vi "Main.vi"() -> ()   [LabVIEW 2015, in "Device Under Test_Cloneable_DQMH.lvlib"]
doc: "This application is based on the Delacor QMH project template. Run this VI directly to test the module in stand alone mode. Run the module tester VI to test the module in external launch mode.\n\nThis example implements a Device Under Test with a cloneable Delacor QMH module.\n_____\nBased on Delacor QMH Project Template 2.0.0.62.\nReviewed and updated to match QMH Project Template 4.0.\n<b>Note:</b> This VI was modified by the <b>Validate DQMH Module</b> tool to upgrade it to the DQMH 3.0 implementation of the 'Show Diagram' message, which checks the password-protected status of the Main VI before showing the diagram.\n____\nDelacor QMH Thermal Chamber Examples 4.0.0.21\nCopyright (c) 2018, Delacor"
uses:
  Device Under Test_Cloneable_DQMH.lvlib
  <vilib>/Delacor/Delacor QMH/Libraries/Cloneable Module Admin_class/Delacor_lib_QMH_Cloneable Module Admin.lvclass
  Module Data--cluster.ctl
  GUI Control References--cluster.ctl
  Set Power State Argument--cluster.ctl
  <vilib>/Delacor/Delacor QMH/Libraries/Cloneable Module Admin_class/Delacor_lib_QMH_Cloneable Module Admin.lvclass/Delacor_lib_QMH_Cloneable Module Admin.ctl
  Perform Self Test Argument--cluster.ctl
  Perform Self Test (Reply Payload)--cluster.ctl
  Update DUT Status Argument--cluster.ctl
  Stop Argument--cluster.ctl
  <vilib>/Delacor/Delacor QMH/Libraries/Module Admin_class/Delacor_lib_QMH_Module Admin.lvclass/Delacor_lib_QMH_Module Admin.ctl
  <vilib>/Delacor/Delacor QMH/Libraries/Cloneable Module Admin_class/Delacor_lib_QMH_Get Module ID.vi
  <vilib>/Delacor/Delacor QMH/Libraries/Module Admin_class/Delacor_lib_QMH_Get External Launch.vi
  <vilib>/Delacor/Delacor QMH/Libraries/Message Queue_class/Delacor_lib_QMH_Enqueue Message (Single).vi
  <vilib>/Utility/error.llb/Error Cluster From Error Code.vi
  <vilib>/ErrorRing/Error Ring.xnode
  <vilib>/Delacor/Delacor QMH/Libraries/Message Queue_class/Delacor_lib_QMH_Message Queue.lvclass
  Clone Registration/Clone Registration.lvlib
panel:
  in  "Self Test":bool
  in  "Power Off":bool
  in  "Power On":bool
  out "Self Test Result":bool
  out "Power  State":bool
  out "error out":errorcluster
  in  "Module Admin":refnum<class "Delacor_lib_QMH_Cloneable Module Admin.lvclass">
  out "Status":string
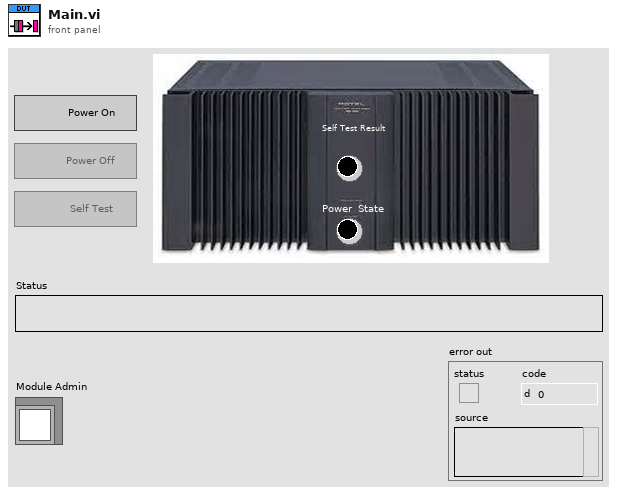
[diagram p1: front panel]
types:
  T1 = typedef "Device Under Test_Cloneable_DQMH.lvlib/Request Events--cluster.ctl" = cluster{"Stop Module":refnum<user-event>, "Show Panel":refnum<user-event>, "Hide Panel":refnum<user-event>, "Show Diagram":refnum<user-event>, "Set Power State":refnum<user-event>, "Perform Self Test":refnum<user-event>, "Update DUT Status":refnum<user-event>, "Get Module Execution Status":refnum<user-event>}
  T2 = typedef "Device Under Test_Cloneable_DQMH.lvlib/Module Data--cluster.ctl" = cluster{"Status":string, "Power State":bool, "Self Test Result":bool, "References":T3}
  T3 = typedef "Device Under Test_Cloneable_DQMH.lvlib/GUI Control References--cluster.ctl" = cluster{"Power On Button":refnum<vi>, "Power Off Button":refnum<vi>, "Self Test Button":refnum<vi>, "Power State LED":refnum<vi>, "Self Test Result LED":refnum<vi>}
  T4 = typedef "Device Under Test_Cloneable_DQMH.lvlib/Set Power State Argument--cluster.ctl" = cluster{"Module ID":i32, "Power State":bool}
  T5 = typedef "Device Under Test_Cloneable_DQMH.lvlib/Perform Self Test Argument--cluster.ctl" = cluster{"Module ID":i32, "Wait Notifier":refnum<notifier>}
  T6 = typedef "Device Under Test_Cloneable_DQMH.lvlib/Update DUT Status Argument--cluster.ctl" = cluster{"Module ID":i32, "Self Test Result":bool, "Power State":bool}
  T7 = enum32{"invalid lock state", "Not Locked", "Locked (No Password)", "Password-protected"}
  T8 = typedef "Device Under Test_Cloneable_DQMH.lvlib/Stop Argument--cluster.ctl" = cluster{"Origin":string, "Module ID":i32, "Exit via Stop Module Req?":bool, "Wait for Module to stop?":bool}
  T9 = enum32{"Invalid", "Standard", "Closed", "Hidden", "Minimized", "Maximized"}
  T10 = typedef "Device Under Test_Cloneable_DQMH.lvlib/Perform Self Test (Reply Payload)--cluster.ctl" = cluster{"Result":bool, "error":errorcluster}
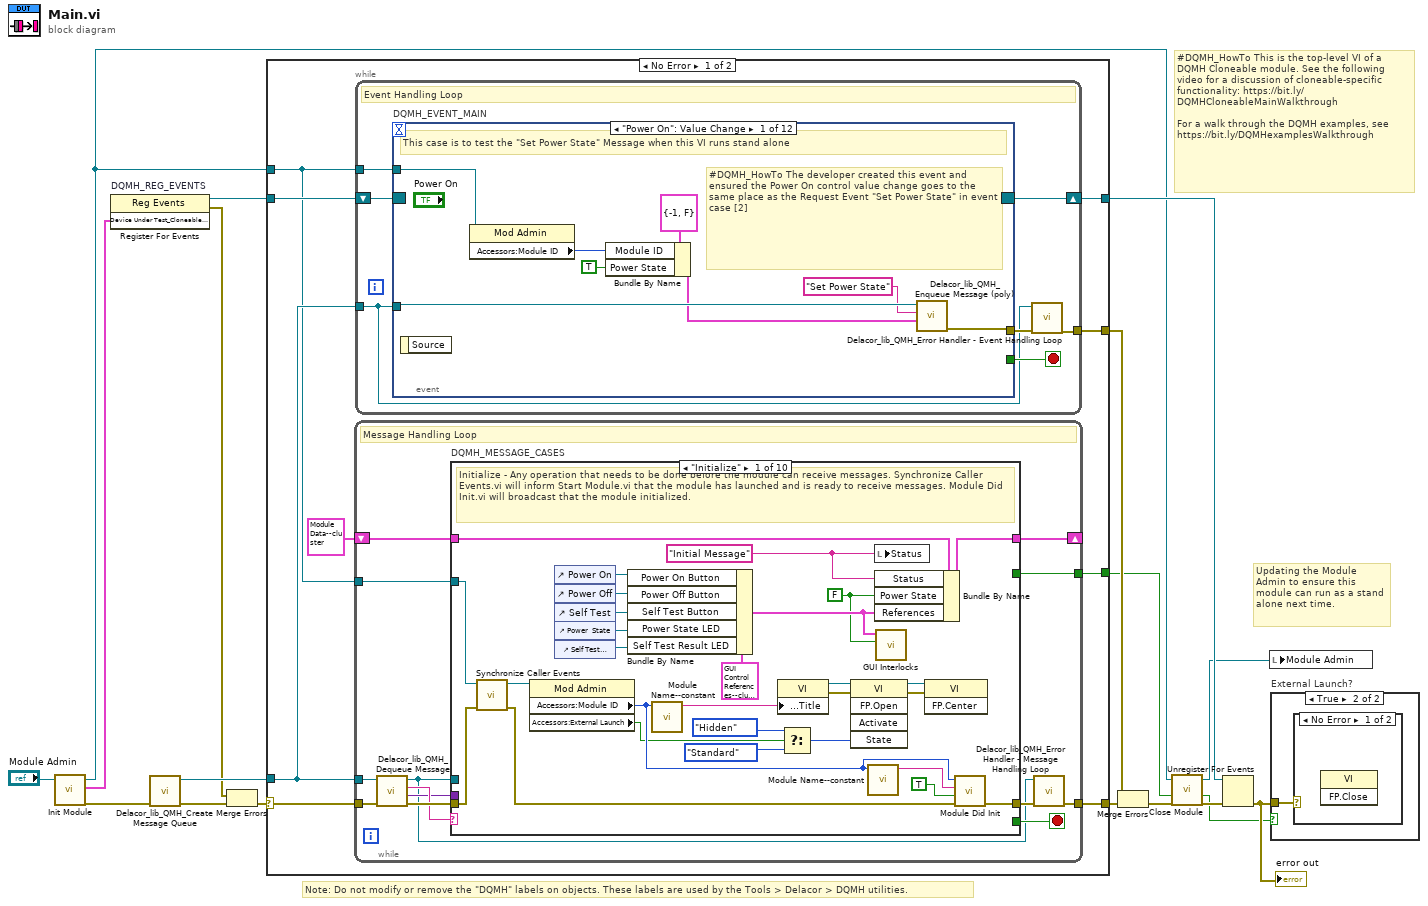
[diagram p0: block diagram]
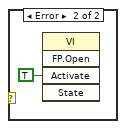
[diagram p3: hidden frame]
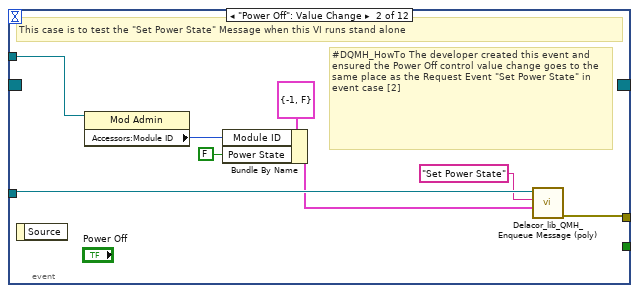
[diagram p4: hidden frame]
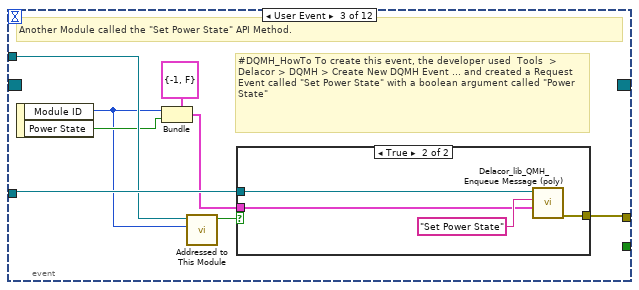
[diagram p5: hidden frame]
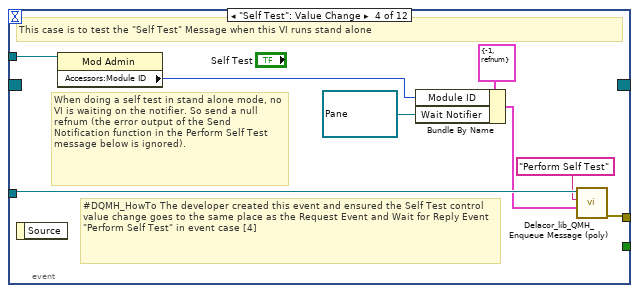
[diagram p7: hidden frame]
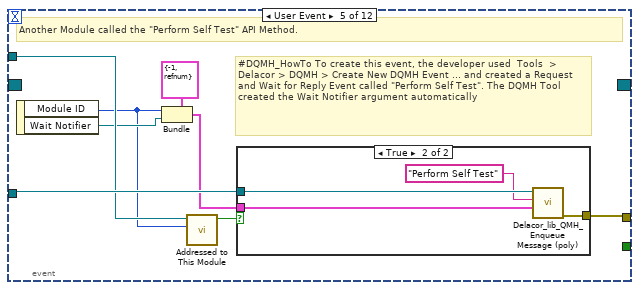
[diagram p8: hidden frame]
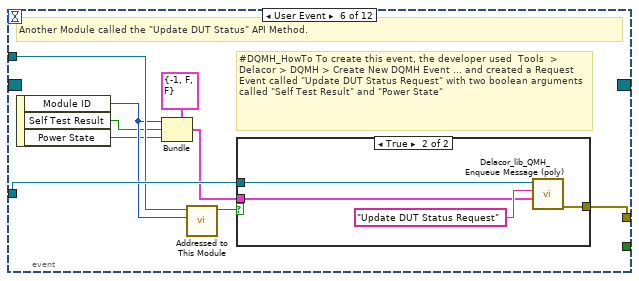
[diagram p10: hidden frame]
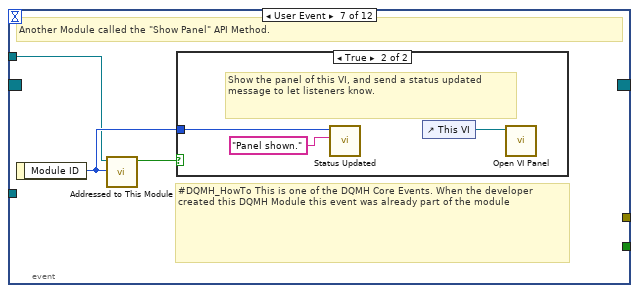
[diagram p12: hidden frame]
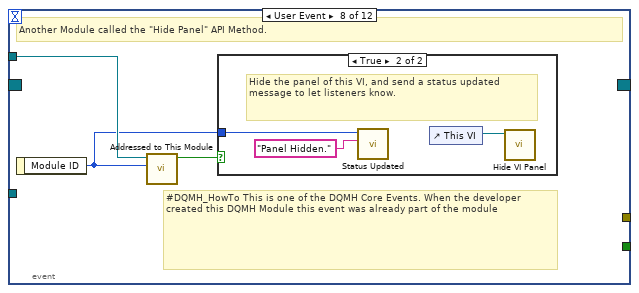
[diagram p14: hidden frame]
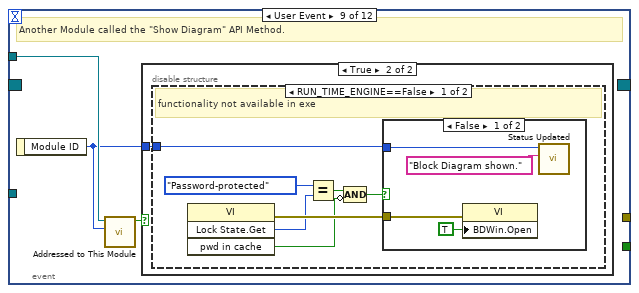
[diagram p16: hidden frame]
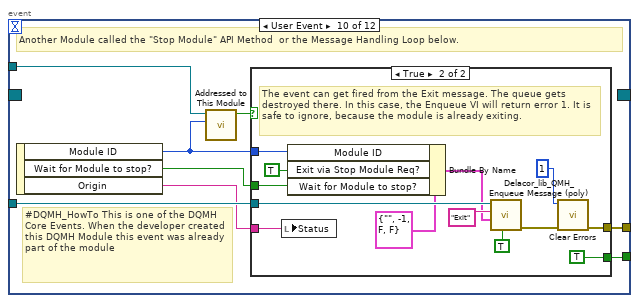
[diagram p20: hidden frame]
diagram:
  # "#DQMH_HowTo This is the top-level VI of a DQMH Cloneable module. See the following video for a discussion of cloneable-specific functionality: https://bit.ly/DQMHCloneableMainWalkthrough\n\nFor a walk through the DQMH examples, see https://bit.ly/DQMHexamplesWalkthrough"
  # "Note: Do not modify or remove the \"DQMH\" labels on objects. These labels are used by the Tools > Delacor > DQMH utilities."
  # "Updating the Module Admin to ensure this module can run as a stand alone next time."
  n1 = call "Init Module.vi"("Cloneable Module Admin in"="Module Admin") -> ("error out"=w15:errorcluster, "Device Under Test_Cloneable_DQMH Request Events"=w12:T1, "Cloneable Module Admin out"=w8:refnum<class "Delacor_lib_QMH_Cloneable Module Admin.lvclass">)  [unwired: 8 in]
  n2 = register-events "DQMH_REG_EVENTS"(w12) -> (reference out=w13:refnum<event-registration>, error out=w1:errorcluster)  [unwired: 2 in]
  n3 = call <vilib>:"Delacor_lib_QMH_Create Message Queue.vi"("error in (no error)"=w15) -> ("error out"=w3:errorcluster, "Message Queue out"=w11:refnum<class "Delacor_lib_QMH_Message Queue.lvclass">)  [unwired: 9 in]
  n4 = Merge Errors(w1, w3) -> (w2:errorcluster)
  n5 = case shown="No Error" w2 {
    selector: w2 -> [w21 w320]
    tunnel: [w27 w320] -> w16
    tunnel: [w26 w321] -> w14
    tunnel: w13 -> [w24 w321]
    tunnel: w11 -> [w23 _]
    tunnel: [w22 _] -> w17
    tunnel: w8 -> [w20 w316]
    tunnel: [w19 _] -> w6
    frame No Error {
      n6 = while {
        tunnel: w23 -> [w165]
        shift-right: [w171] -> _
        shift-left: T2 {"Status"="", "Power State"=FALSE, "Self Test Result"=FALSE, "References"={"Power On Button"=refnum, "Power Off Button"=refnum, "Self Test Button"=refnum, "Power State LED"=refnum, "Self Test Result LED"=refnum}} ("Data Cluster") -> [w172]
        tunnel: w21 -> [w169]
        tunnel: [w163] -> w27
        tunnel: w20 -> [w162]
        tunnel: [w161] -> w19
        stop <- w170 stop-if-true
        # "Message Handling Loop"
        n7 = call-dynamic "Delacor_lib_QMH_Dequeue Message.vi"("error in (no error)"=w169, "Message Queue in"=w165) -> ("error out"=w168:errorcluster, "Message Data"=w166:variant, "Message"=w167:string, "Message Queue out"=w164:refnum<class "Delacor_lib_QMH_Message Queue.lvclass">)  [unwired: 6 in]
        n8 = case "DQMH_MESSAGE_CASES" shown="\"Initialize\"" w167 {
          selector: w167 -> [_ _ _ _ _ _ _ _ _ w303]
          tunnel: w164 -> [_ _ _ w228 w239 w251 _ w267 w297 _]
          tunnel: w168 -> [w193 w214 w216 w230 w246 w264 w266 w277 w299 _]
          tunnel: [w186 w206 w216 w220 w231 w252 w266 w272 w293 w304] -> w173
          tunnel: w172 -> [w192 w205 w215 w227 w235 w263 w265 w276 w296 w305]
          tunnel: [w191 w205 w215 w224 w242 w263 w265 w276 w296 w305] -> w171
          tunnel: [_ _ _ _ _ _ _ _ w295 _] -> w170
          tunnel: w166 -> [_ w213 _ w217 w238 w262 _ w275 w289 _]
          tunnel: w162 -> [w183 w209 _ _ _ _ _ w271 w285 w301]
          tunnel: [_ _ _ _ _ _ _ _ w287 _] -> w161
          frame "Initialize" {
            w174 = FALSE ("Power State")
            w190 = "Initial Message" ("Initial Message")
            # "Initialize - Any operation that needs to be done before the module can receive messages. Synchronize Caller Events.vi will inform Start Module.vi that the module has launched and is ready to receive messages. Module Did Init.vi will broadcast that the module initialized."
            n9 = call "Synchronize Caller Events.vi"("error in (no error)"=w193, "Module Admin"=w183) -> ("error out"=w187:errorcluster, "Module Admin out"=w182:refnum<class "Delacor_lib_QMH_Cloneable Module Admin.lvclass">)  [unwired: 8 in]
            n10 = property class="Mod Admin"(reference=w182) -> ("Accessors:Module ID"=w185:i32, "Accessors:External Launch"=w184:bool)  [unwired: 1 in, 2 out]
            n11 = control-ref of="Power On"() -> (w180:refnum<vi>)
            n12 = control-ref of="Power Off"() -> (w179:refnum<vi>)
            n13 = control-ref of="Self Test"() -> (w178:refnum<vi>)
            n14 = control-ref of="Power  State"() -> (w177:refnum<vi>)
            n15 = control-ref of="Self Test Result"() -> (w176:refnum<vi>)
            n16 = Bundle By Name(cluster=T3 {"Power On Button"=refnum, "Power Off Button"=refnum, "Self Test Button"=refnum, "Power State LED"=refnum, "Self Test Result LED"=refnum} ("References"), "Power On Button"=w180, "Power Off Button"=w179, "Self Test Button"=w178, "Power State LED"=w177, "Self Test Result LED"=w176) -> (w175:T3)
            n17 = call "Module Name--constant.vi"("Module ID"=w185) -> ("Module Name"=w197:string)  [unwired: 10 in]
            n18 = property class="VI"("Front Panel.Title"=w197) -> (reference out=w200:refnum<vi>, error out=w201:errorcluster)  [unwired: 2 in]
            n19 = Select(t=T9."Hidden" ("State"), s=w184, f=T9."Standard" ("State")) -> (s? t:f=w194:T9)
            n20 = invoke class="VI" method="FP.Open"(reference=w200, error in=w201, "State"=w194) -> (reference out=w199:refnum<vi>, error out=w198:errorcluster)  [unwired: 2 in, 3 out]
            n21 = call "Module Name--constant.vi"("Module ID"=w185) -> ("Module Name"=w188:string)  [unwired: 10 in]
            n22 = local write "Status"(w190) -> ()
            n23 = Bundle By Name(cluster=w192, "Status"=w190, "Power State"=w174, "References"=w175) -> (w191:T2)
            n24 = call "GUI Interlocks.vi"("Power State"=w174, "References"=w175) -> ()  [unwired: 10 in]
            n25 = invoke class="VI" method="FP.Center"(reference=w199, error in=w198) -> ()  [unwired: 1 in, 3 out]
            n26 = call "Module Did Init.vi"("error in (no error)"=w187, "Initialized?"=TRUE, "Origin"=w188, "Module ID"=w185) -> ("error out"=w186:errorcluster)  [unwired: 7 in]
          }
          frame "Update Display" {
            # "Update Display - Update user interface here."
            n27 = property class="Mod Admin"(reference=w209) -> ("Accessors:Module ID"=w208:i32)  [unwired: 1 in, 2 out]
            n28 = Variant To Data(error in=w214, type="", Variant=w213) -> (data=w211:string, error out=w210:errorcluster)
            "Status" <- w211
            n29 = Unbundle By Name(w205) -> ("References"=w204:T3, "Power State"=w203:bool, "Self Test Result"=w202:bool)
            "Power  State" <- w203
            "Self Test Result" <- w202
            n30 = call "Status Updated.vi"("error in (no error)"=w210, "Status"=w211, "Module ID"=w208) -> ("error out"=w207:errorcluster)  [unwired: 8 in]
            n31 = call "GUI Interlocks.vi"("Power State"=w203, "References"=w204) -> ()  [unwired: 10 in]
            n32 = call "DUT Status Updated.vi"("error in (no error)"=w207, "Self Test Result"=w202, "Power State"=w203, "Module ID"=w208) -> ("error out"=w206:errorcluster)  [unwired: 7 in]
          }
          frame "---DUT---" {
            # "Separator - The following cases handle DUT specific messages."
          }
          frame "Set Power State" {
            # "#DQMH_HowTo To create this case, the developer used  Tools  > Delacor > DQMH > Create New DQMH Event ... and created a Request Event called \"Set Power State\" with a boolean argument called \"Power State\""
            # "Update the power state of the DUT. Broadcast a message that the power state was updated."
            n33 = Variant To Data(error in=w230, type=T4 {"Module ID"=-1, "Power State"=FALSE} ("Set Power State Argument"), Variant=w217) -> (data=w225:T4, error out=w229:errorcluster)
            n34 = Unbundle By Name(w225) -> ("Power State"=w219:bool)
            n35 = Format Into String(format string="DUT Power State Set to %s", w219) -> (resulting string=w221:string)  [unwired: 2 in, 1 out]
            n36 = Bundle By Name(cluster=w227, "Power State"=w219, "Self Test Result"=FALSE) -> (w224:T2)
            n37 = call-poly <vilib>:"Delacor_lib_QMH_Enqueue Message (poly).vi"("error in (no error)"=w229, "Message Data"=w221, "Message"="Update Display", "Message Queue in"=w228) -> ("error out"=w220:errorcluster)  [unwired: 6 in, 1 out]
          }
          frame "Perform Self Test" {
            # "#DQMH_HowTo To create this case, the developer used  Tools  > Delacor > DQMH > Create New DQMH Event ... and created a Request Event and Wait for Reply called \"Perform Self Test\" without arguments"
            # "Perform a self test of the DUT. Update the display with the result, and broadcast a message indicating the result of the self test."
            n38 = Unbundle By Name(w235) -> ("Power State"=w234:bool)
            n39 = Variant To Data(error in=w246, type=T5 {"Module ID"=-1, "Wait Notifier"=refnum} ("Perform Self Test Argument"), Variant=w238) -> (data=w244:T5, error out=w232:errorcluster)
            n40 = Unbundle By Name(w244) -> ("Wait Notifier"=w243:refnum<notifier>)
            n41 = case shown="True" w234 {
              tunnel: [_ w249] -> w236
              tunnel: ["DUT is powered off, cannot perform self test." ("format string") w248] -> w233
              frame False {
              }
              frame True {
                n42 = call "Simulate Self Test.vi"() -> ("Result"=w249:bool)  [unwired: 11 in]
                n43 = Format Into String(format string="DUT Self Test Result: %s", w249) -> (resulting string=w248:string)  [unwired: 2 in, 1 out]
              }
            }
            n44 = Bundle By Name(cluster=T10 {"Result"=FALSE, "error"={"status"=FALSE, "code"=0, "source"=""}} ("notification"), "Result"=w236, "error"=w232) -> (w240:T10)
            n45 = Bundle By Name(cluster=w235, "Self Test Result"=w236) -> (w242:T2)
            n46 = Send Notification(notification=w240, notifier=w243) -> ()  [unwired: 1 in, 2 out]
            n47 = call-poly <vilib>:"Delacor_lib_QMH_Enqueue Message (poly).vi"("error in (no error)"=w232, "Message Data"=w233, "Message"="Update Display", "Message Queue in"=w239) -> ("error out"=w231:errorcluster)  [unwired: 6 in, 1 out]
          }
          frame "Update DUT Status Request" {
            # "#DQMH_HowTo To create this case, the developer used  Tools  > Delacor > DQMH > Create New DQMH Event ... and created a Request Event called \"Update DUT Status Request\" with two boolean arguments called \"Self Test Result\" and \"Power State\""
            # "Read the state of the DUT and broadcast it."
            n48 = Variant To Data(error in=w264, type=T6 {"Module ID"=-1, "Self Test Result"=FALSE, "Power State"=FALSE} ("Update DUT Status Request Argument"), Variant=w262) -> (data=w260:T6, error out=w256:errorcluster)
            n49 = Unbundle By Name(w260) -> ("Module ID"=w259:i32, "Self Test Result"=w258:bool, "Power State"=w257:bool)
            n50 = call "DUT Status Updated.vi"("error in (no error)"=w256, "Self Test Result"=w257, "Power State"=w258, "Module ID"=w259) -> ("error out"=w253:errorcluster)  [unwired: 7 in]
            n51 = call-poly <vilib>:"Delacor_lib_QMH_Enqueue Message (poly).vi"("error in (no error)"=w253, "Message Data"="DUT Status Updated" ("format string"), "Message"="Update Display", "Message Queue in"=w251) -> ("error out"=w252:errorcluster)  [unwired: 6 in, 1 out]
          }
          frame "---Exit and Error Handling---" {
            # "Separator - The following cases handle error and exit messages."
          }
          frame "Error" {
            # "#DQMH_HowTo When the developer created this DQMH Module this case was already part of the module"
            # "Error - Check the error message data and respond accordingly. This message is sent by the \"Error Handler\" VIs at the end of each loop in this application."
            n52 = property class="Mod Admin"(reference=w271) -> ("Accessors:External Launch"=w268:bool, "Accessors:Module ID"=w270:i32)  [unwired: 1 in, 2 out]
            n53 = Variant To Data(error in=w277, type=errorcluster {"status"=FALSE, "code"=0, "source"=""} ("error constant"), Variant=w275) -> (data=w278:errorcluster, error out=w273:errorcluster)
            n54 = call "Error Reported.vi"("Error"=w278, "Module ID"=w270) -> ()  [unwired: 9 in, 1 out]
            n55 = case shown="False" w268 {
              tunnel: [w283 _] -> w269
              tunnel: w267 -> [w282 _]
              tunnel: w278 -> [w279 _]
              frame False {
                # "If the module is running standalone, then pop up an error dialog and call the \"Exit\" message."
                n56 = call <vilib>:"Simple Error Handler.vi"("error in (no error)"=w279) -> ()  [unwired: 4 in, 5 out]
                n57 = call-poly <vilib>:"Delacor_lib_QMH_Enqueue Message (poly).vi"("Priority Message? (F)"=TRUE, "Message"="Exit", "Message Queue in"=w282) -> ("error out"=w283:errorcluster)  [unwired: 7 in, 1 out]
              }
              frame True {
                # "If the module was launched externally, calling the Error Reported broadcast VI is the only action performed by the \"Error\" message. The module's caller can then process the error appropriately."
              }
            }
            n58 = Merge Errors(w273, w269) -> (w272:errorcluster)
          }
          frame "Exit" {
            w291 = 91  # 91: not all Exit messages will have an argument
            w295 = TRUE  # Stop the VI
            # "#DQMH_HowTo When the developer created this DQMH Module this case was already part of the module"
            # "Release the message queue reference"
            # "Exit - Exit the application."
            n59 = Variant To Data(error in=w299, type=T8 {"Origin"="", "Module ID"=-1, "Exit via Stop Module Req?"=FALSE, "Wait for Module to stop?"=FALSE} ("Stop Argument"), Variant=w289) -> (data=w286:T8, error out=w290:errorcluster)
            n60 = call <vilib>:"Clear Errors.vi"("error in (no error)"=w290, "specific error code to clear (0: all)"=w291) -> ("error out"=w298:errorcluster)  [unwired: 4 in, 1 out]
            n61 = control-ref of="This VI"() -> (w284:refnum<vi>)
            n62 = call-dynamic "Delacor_lib_QMH_Release Message Queue.vi"("error in (no error)"=w298, "Message Queue"=w297) -> ("error out"=w294:errorcluster)  [unwired: 9 in]
            n63 = call "Handle Exit.vi"("Stop Argument"=w286, "Module Admin in"=w285, "VI reference"=w284) -> ("error out"=w292:errorcluster, "Wait for Stop?"=w287:bool)  [unwired: 7 in]
            n64 = Merge Errors(w292, w294) -> (w293:errorcluster)
          }
          frame Default {
            # "#DQMH_HowTo When the developer created this DQMH Module this case was already part of the module"
            # "'Default' case only runs if there is a message that isn't defined in any of the other cases.  Output a programming error."
            n65 = property class="Mod Admin"(reference=w301) -> ("Accessors:Module ID"=w300:i32)  [unwired: 1 in, 2 out]
            n66 = call "Module Name--constant.vi"("Module ID"=w300) -> ("Module Name"=w302:string)  [unwired: 10 in]
            n67 = xnode "Error Ring"("parameter 0"=w303, "parameter 1"=w302) -> ("error out"=w304:errorcluster)
          }
        }
        n68 = call-dynamic "Delacor_lib_QMH_Error Handler - Message Handling Loop.vi"("error in (no error)"=w173, "Message Queue in"=w164) -> ("dup error in"=w163:errorcluster)  [unwired: 8 in, 1 out]
      }
      n69 = while {
        tunnel: w23 -> [w28]
        shift-right: [w33] -> w26
        shift-left: w24 -> [w34]
        tunnel: [w30] -> w22
        tunnel: w20 -> [w29]
        stop <- w31 stop-if-true
        # "Event Handling Loop"
        n70 = event "DQMH_EVENT_MAIN" shown="[0] \"Power On\": Value Change" {
          selector: w34 -> [_ _ _ _ _ _ _ _ _ _ _ _]
          dyn-events: [_ _ _ _ _ _ _ _ _ _ _ _] -> w33
          timeout: _ -> [_ _ _ _ _ _ _ _ _ _ _ _]
          tunnel: [_ _ _ _ _ _ _ _ _ w126 _ _] -> w31
          tunnel: w28 -> [w42 w50 w58 w70 w78 w91 _ _ _ w129 w144 _]
          tunnel: [w39 w47 w53 w66 w73 w86 _ _ _ w130 w146 w154] -> w32
          tunnel: w29 -> [w37 w45 w56 w69 w76 w89 w96 w103 w110 w128 w147 w156]
          event "Power On": Value Change {
            # "#DQMH_HowTo The developer created this event and ensured the Power On control value change goes to the same place as the Request Event \"Set Power State\" in event case [2]"
            # "This case is to test the \"Set Power State\" Message when this VI runs stand alone"
            n71 = event-data() -> ()  [unwired: 1 in, 1 out]
            n72 = property class="Mod Admin"(reference=w37) -> ("Accessors:Module ID"=w36:i32)  [unwired: 1 in, 2 out]
            n73 = Bundle By Name(cluster=T4 {"Module ID"=-1, "Power State"=FALSE} ("Set Power State Argument"), "Module ID"=w36, "Power State"=TRUE) -> (w40:T4)
            n74 = call-poly <vilib>:"Delacor_lib_QMH_Enqueue Message (poly).vi"("Message Data"=w40, "Message"="Set Power State", "Message Queue in"=w42) -> ("error out"=w39:errorcluster)  [unwired: 7 in, 1 out]
          }
          event "Power Off": Value Change {
            # "#DQMH_HowTo The developer created this event and ensured the Power Off control value change goes to the same place as the Request Event \"Set Power State\" in event case [2]"
            # "This case is to test the \"Set Power State\" Message when this VI runs stand alone"
            n75 = event-data() -> ()  [unwired: 1 in, 1 out]
            n76 = property class="Mod Admin"(reference=w45) -> ("Accessors:Module ID"=w44:i32)  [unwired: 1 in, 2 out]
            n77 = Bundle By Name(cluster=T4 {"Module ID"=-1, "Power State"=FALSE} ("Set Power State Argument"), "Module ID"=w44, "Power State"=FALSE) -> (w48:T4)
            n78 = call-poly <vilib>:"Delacor_lib_QMH_Enqueue Message (poly).vi"("Message Data"=w48, "Message"="Set Power State", "Message Queue in"=w50) -> ("error out"=w47:errorcluster)  [unwired: 7 in, 1 out]
          }
          event User Event {
            # "#DQMH_HowTo To create this event, the developer used  Tools  > Delacor > DQMH > Create New DQMH Event ... and created a Request Event called \"Set Power State\" with a boolean argument called \"Power State\""
            # "Another Module called the \"Set Power State\" API Method."
            n79 = event-data() -> ("Module ID"=w51:i32, "Power State"=w52:bool)  [unwired: 1 in]
            n80 = Bundle(cluster=T4 {"Module ID"=-1, "Power State"=FALSE} ("Set Power State Argument"), "Module ID"=w51, "Power State"=w52) -> (w54:T4)
            n81 = call "Addressed to This Module.vi"("Module ID from Argument"=w51, "Module Admin"=w56) -> ("Addressed to this instance?"=w57:bool)  [unwired: 8 in, 1 out]
            n82 = case shown="True" w57 {
              tunnel: w58 -> [_ w62]
              tunnel: w54 -> [_ w60]
              tunnel: [_ w59] -> w53
              frame False {
              }
              frame True {
                n83 = call-poly <vilib>:"Delacor_lib_QMH_Enqueue Message (poly).vi"("Message Data"=w60, "Message"="Set Power State", "Message Queue in"=w62) -> ("error out"=w59:errorcluster)  [unwired: 7 in, 1 out]
              }
            }
          }
          event "Self Test": Value Change {
            # "#DQMH_HowTo The developer created this event and ensured the Self Test control value change goes to the same place as the Request Event and Wait for Reply Event \"Perform Self Test\" in event case [4]"
            # "When doing a self test in stand alone mode, no VI is waiting on the notifier. So send a null refnum (the error output of the Send Notification function in the Perform Self Test message below is ignored)."
            # "This case is to test the \"Self Test\" Message when this VI runs stand alone"
            n84 = event-data() -> ()  [unwired: 1 in, 1 out]
            n85 = property class="Mod Admin"(reference=w69) -> ("Accessors:Module ID"=w63:i32)  [unwired: 1 in, 2 out]
            n86 = Bundle By Name(cluster=T5 {"Module ID"=-1, "Wait Notifier"=refnum} ("Perform Self Test Argument"), "Module ID"=w63, "Wait Notifier"=refnum<notifier> refnum) -> (w67:T5)
            n87 = call-poly <vilib>:"Delacor_lib_QMH_Enqueue Message (poly).vi"("Message Data"=w67, "Message"="Perform Self Test", "Message Queue in"=w70) -> ("error out"=w66:errorcluster)  [unwired: 7 in, 1 out]
          }
          event User Event {
            # "#DQMH_HowTo To create this event, the developer used  Tools  > Delacor > DQMH > Create New DQMH Event ... and created a Request and Wait for Reply Event called \"Perform Self Test\". The DQMH Tool created the Wait Notifier argument automatically"
            # "Another Module called the \"Perform Self Test\" API Method."
            n88 = event-data() -> ("Module ID"=w71:i32, "Wait Notifier"=w72:refnum<notifier>)  [unwired: 1 in]
            n89 = Bundle(cluster=T5 {"Module ID"=-1, "Wait Notifier"=refnum} ("Perform Self Test Argument"), "Module ID"=w71, "Wait Notifier"=w72) -> (w74:T5)
            n90 = call "Addressed to This Module.vi"("Module ID from Argument"=w71, "Module Admin"=w76) -> ("Addressed to this instance?"=w77:bool)  [unwired: 8 in, 1 out]
            n91 = case shown="True" w77 {
              tunnel: w78 -> [_ w82]
              tunnel: w74 -> [_ w80]
              tunnel: [_ w79] -> w73
              frame False {
              }
              frame True {
                n92 = call-poly <vilib>:"Delacor_lib_QMH_Enqueue Message (poly).vi"("Message Data"=w80, "Message"="Perform Self Test", "Message Queue in"=w82) -> ("error out"=w79:errorcluster)  [unwired: 7 in, 1 out]
              }
            }
          }
          event User Event {
            # "#DQMH_HowTo To create this event, the developer used  Tools  > Delacor > DQMH > Create New DQMH Event ... and created a Request Event called \"Update DUT Status Request\" with two boolean arguments called \"Self Test Result\" and \"Power State\""
            # "Another Module called the \"Update DUT Status\" API Method."
            n93 = event-data() -> ("Module ID"=w85:i32, "Self Test Result"=w84:bool, "Power State"=w83:bool)  [unwired: 1 in]
            n94 = Bundle(cluster=T6 {"Module ID"=-1, "Self Test Result"=FALSE, "Power State"=FALSE} ("Update DUT Status Request Argument"), "Module ID"=w85, "Self Test Result"=w84, "Power State"=w83) -> (w87:T6)
            n95 = call "Addressed to This Module.vi"("Module ID from Argument"=w85, "Module Admin"=w89) -> ("Addressed to this instance?"=w90:bool)  [unwired: 8 in, 1 out]
            n96 = case shown="True" w90 {
              tunnel: w91 -> [_ w95]
              tunnel: w87 -> [_ w93]
              tunnel: [_ w92] -> w86
              frame False {
              }
              frame True {
                n97 = call-poly <vilib>:"Delacor_lib_QMH_Enqueue Message (poly).vi"("Message Data"=w93, "Message"="Update DUT Status Request", "Message Queue in"=w95) -> ("error out"=w92:errorcluster)  [unwired: 7 in, 1 out]
              }
            }
          }
          event User Event {
            # "#DQMH_HowTo This is one of the DQMH Core Events. When the developer created this DQMH Module this event was already part of the module"
            # "Another Module called the \"Show Panel\" API Method."
            n98 = event-data() -> ("Module ID"=w97:i32)  [unwired: 1 in]
            n99 = call "Addressed to This Module.vi"("Module ID from Argument"=w97, "Module Admin"=w96) -> ("Addressed to this instance?"=w98:bool)  [unwired: 8 in, 1 out]
            n100 = case shown="True" w98 {
              tunnel: w97 -> [_ w100]
              frame False {
              }
              frame True {
                # "Show the panel of this VI, and send a status updated message to let listeners know."
                n101 = call "Status Updated.vi"("Status"="Panel shown." ("format string"), "Module ID"=w100) -> ()  [unwired: 9 in, 1 out]
                n102 = control-ref of="This VI"() -> (w99:refnum<vi>)
                n103 = call "Open VI Panel.vi"("VI"=w99) -> ()  [unwired: 10 in, 1 out]
              }
            }
          }
          event User Event {
            # "#DQMH_HowTo This is one of the DQMH Core Events. When the developer created this DQMH Module this event was already part of the module"
            # "Another Module called the \"Hide Panel\" API Method."
            n104 = event-data() -> ("Module ID"=w102:i32)  [unwired: 1 in]
            n105 = call "Addressed to This Module.vi"("Module ID from Argument"=w102, "Module Admin"=w103) -> ("Addressed to this instance?"=w104:bool)  [unwired: 8 in, 1 out]
            n106 = case shown="True" w104 {
              tunnel: w102 -> [_ w106]
              frame False {
              }
              frame True {
                # "Hide the panel of this VI, and send a status updated message to let listeners know."
                n107 = call "Status Updated.vi"("Status"="Panel Hidden.", "Module ID"=w106) -> ()  [unwired: 9 in, 1 out]
                n108 = control-ref of="This VI"() -> (w105:refnum<vi>)
                n109 = call "Hide VI Panel.vi"("VI"=w105) -> ()  [unwired: 10 in, 1 out]
              }
            }
          }
          event User Event {
            # "Another Module called the \"Show Diagram\" API Method."
            n110 = event-data() -> ("Module ID"=w109:i32)  [unwired: 1 in]
            n111 = call "Addressed to This Module.vi"("Module ID from Argument"=w109, "Module Admin"=w110) -> ("Addressed to this instance?"=w108:bool)  [unwired: 8 in, 1 out]
            n112 = case shown="True" w108 {
              tunnel: w109 -> [_ w111]
              frame False {
                # "#DQMH_HowTo This is one of the DQMH Core Events. When the developer created this DQMH Module this event was already part of the module"
              }
              frame True {
                n113 = disable-structure shown="RUN_TIME_ENGINE==False" {
                  disable-tunnel: w111 -> [w112 _]
                  frame condition #0 (active) {
                    # "functionality not available in exe"
                    n114 = invoke class="VI" method="Lock State.Get"() -> (error out=w118:errorcluster, "Get Lock State"=w117:T7, "pwd in cache"=w114:bool)  [unwired: 4 in, 1 out]
                    n115 = Equal?(x=T7."Password-protected", y=w117) -> (x = y?=w115:bool)
                    n116 = Compound Arithmetic op=AND(w115, invert w114) -> (w113:bool)
                    n117 = case shown="False" w113 {
                      tunnel: w118 -> [w121 _]
                      tunnel: w112 -> [w119 _]
                      frame False {
                        n118 = property class="VI"(error in=w121, "BDWin.Open"=TRUE ("Block Diagram Window:Open")) -> ()  [unwired: 1 in, 2 out]
                        n119 = call "Status Updated.vi"("Status"="Block Diagram shown." ("format string"), "Module ID"=w119) -> ()  [unwired: 9 in, 1 out]
                      }
                      frame True {
                        # "Password-protected VI, and the password is not in the cache. Do not show the diagram."
                      }
                    }
                  }
                  frame condition #1 {
                  }
                }
              }
            }
          }
          event User Event {
            # "#DQMH_HowTo This is one of the DQMH Core Events. When the developer created this DQMH Module this event was already part of the module"
            # "Another Module called the \"Stop Module\" API Method  or the Message Handling Loop below."
            n120 = event-data() -> ("Module ID"=w124:i32, "Wait for Module to stop?"=w125:bool, "Origin"=w123:string)  [unwired: 1 in]
            n121 = call "Addressed to This Module.vi"("Module ID from Argument"=w124, "Module Admin"=w128) -> ("Addressed to this instance?"=w127:bool)  [unwired: 8 in, 1 out]
            n122 = case shown="True" w127 {
              tunnel: [_ w139] -> w130
              tunnel: w129 -> [_ w138]
              tunnel: [_ TRUE] -> w126
              tunnel: w125 -> [_ w133]
              tunnel: w124 -> [_ w135]
              tunnel: w123 -> [_ w131]
              frame False {
              }
              frame True {
                # "The event can get fired from the Exit message. The queue gets destroyed there. In this case, the Enqueue VI will return error 1. It is safe to ignore, because the module is already exiting."
                n123 = local write "Status"(w131) -> ()
                n124 = Bundle By Name(cluster=T8 {"Origin"="", "Module ID"=-1, "Exit via Stop Module Req?"=FALSE, "Wait for Module to stop?"=FALSE} ("Stop Argument"), "Module ID"=w135, "Exit via Stop Module Req?"=TRUE, "Wait for Module to stop?"=w133) -> (w132:T8)
                n125 = call-poly <vilib>:"Delacor_lib_QMH_Enqueue Message (poly).vi"("Priority Message? (F)"=TRUE, "Message Data"=w132, "Message"="Exit", "Message Queue in"=w138) -> ("error out"=w142:errorcluster)  [unwired: 6 in, 1 out]
                n126 = call <vilib>:"Clear Errors.vi"("error in (no error)"=w142, "specific error code to clear (0: all)"=1) -> ("error out"=w139:errorcluster)  [unwired: 4 in, 1 out]
              }
            }
          }
          event Panel Close? {
            w148 = TRUE  # Discard the event so the Exit message has a chance to run.
            # "#DQMH_HowTo When the developer created this DQMH Module this event was already part of the module"
            # "Send the Exit message if the user closes the panel of the VI."
            n127 = event-data() -> ()  [unwired: 1 in, 1 out]
            n128 = property class="Mod Admin"(reference=w147) -> ("Accessors:External Launch"=w145:bool)  [unwired: 1 in, 2 out]
            n129 = case shown="False" w145 {
              tunnel: w144 -> [_ w153]
              tunnel: [_ w152] -> w146
              frame True {
                # "If externally launched, clicking the 'X' hides the panel, but doesn't close it."
                n130 = control-ref of="This VI"() -> (w149:refnum<vi>)
                n131 = call "Hide VI Panel.vi"("VI"=w149) -> ()  [unwired: 10 in, 1 out]
              }
              frame False {
                # "If run as a stand-alone VI, clicking the panel 'X' stops the VI."
                n132 = call-poly <vilib>:"Delacor_lib_QMH_Enqueue Message (poly).vi"("Priority Message? (F)"=TRUE, "Message"="Exit", "Message Queue in"=w153) -> ("error out"=w152:errorcluster)  [unwired: 7 in, 1 out]
              }
            }
            n133 = event-data("Discard?"=w148) -> ()  [unwired: 1 in, 1 out]
          }
          event User Event {
            # "#DQMH_HowTo This is one of the DQMH Core Events. When the developer created this DQMH Module this event was already part of the module"
            # "For cloneable running as singleton, broadcast that the module is running."
            n134 = event-data() -> ("Module ID"=w155:i32)  [unwired: 1 in]
            n135 = call "Addressed to This Module.vi"("Module ID from Argument"=w155, "Module Admin"=w156) -> ("Addressed to this instance?"=w157:bool)  [unwired: 8 in, 1 out]
            n136 = case shown="True" w157 {
              tunnel: w155 -> [_ w160]
              tunnel: [_ w158] -> w154
              frame False {
              }
              frame True {
                n137 = call "Update Module Execution Status.vi"("Running?"=TRUE, "Module ID"=w160) -> ("error out"=w158:errorcluster)  [unwired: 9 in]
              }
            }
          }
        }
        n138 = call-dynamic "Delacor_lib_QMH_Error Handler - Event Handling Loop.vi"("error in (no error)"=w32, "Message Queue in"=w28) -> ("dup error in"=w30:errorcluster)  [unwired: 8 in, 1 out]
      }
    }
    frame Error {
      n139 = call "Synchronize Caller Events.vi"("Module Admin"=w316) -> ("Module Admin out"=w315:refnum<class "Delacor_lib_QMH_Cloneable Module Admin.lvclass">)  [unwired: 9 in, 1 out]
      n140 = property class="Mod Admin"(reference=w315) -> ("Accessors:Module ID"=w314:i32)  [unwired: 1 in, 2 out]
      n141 = call "Module Name--constant.vi"("Module ID"=w314) -> ("Module Name"=w319:string)  [unwired: 10 in]
      n142 = call "Remove.vi"("Module ID"=w314) -> ()  [unwired: 9 in, 2 out]
      n143 = Format Into String(format string="An error occurred during initialization. %s is no longer running.", w319) -> (resulting string=w317:string)  [unwired: 2 in, 1 out]
      n144 = call "Error Reported.vi"("Additional Information"=w317, "Error"=w320, "Module ID"=w314) -> ()  [unwired: 8 in, 1 out]
    }
  }
  n145 = Merge Errors(w17, w16) -> (w18:errorcluster)
  n146 = call "Close Module.vi"("error in (no error)"=w18, "Wait for stop?"=w6, "Module Admin in"=w8) -> ("error out"=w10:errorcluster, "External Launch"=w4:bool, "Module Admin out"=w7:refnum<class "Delacor_lib_QMH_Cloneable Module Admin.lvclass">)  [unwired: 6 in]
  n147 = Unregister For Events(event registration refnum=w14, error in=w10) -> (error out=w5:errorcluster)
  "error out" <- w5
  n148 = local write "Module Admin"(w7) -> ()
  n149 = case "External Launch?" shown="True" w4 {
    tunnel: w5 -> [_ w322]
    frame False {
    }
    frame True {
      n150 = case shown="No Error" w322 {
        frame No Error {
          n151 = invoke class="VI" method="FP.Close"() -> ()  [unwired: 3 in, 3 out]
        }
        frame Error {
          n152 = invoke class="VI" method="FP.Open"("Activate"=TRUE ("Activate?")) -> ()  [unwired: 4 in, 5 out]
        }
      }
    }
  }
